vi "RunningAverage-AddResultChannels.vi"(8 "Error in":errorcluster, 10 "CD Settings in":T1 {"CD Task Dependency Ref" format="%.0x"; "CD Task Dependency" format="%.0x"}, 11 "Custom Device ref":T2 format="%.0x") -> (0 "Error out":errorcluster, 3 "Custom Device ref out":T2 format="%.0x")   [LabVIEW 2017, in "Waveform-Processing-Custom-Device Shared.lvlib" / "Running Average.lvlib"]
uses:
  Running Average.lvlib
  <vilib>/NI Veristand/Custom Device API/Custom Device Item Ref.ctl
  Custom Device Settings.ctl
  <vilib>/NI Veristand/Custom Device API/Custom Device Channel.ctl
  <vilib>/NI Veristand/Custom Device API/Custom Device Channel Type.ctl
  NationalInstruments.VeriStand.SystemStorage
  Constants.vi
  <vilib>/NI Veristand/Custom Device API/Get Item Property (Dependent Node Pointer).vi
  <vilib>/NI Veristand/Custom Device API/Set Item Property (Dependent Node Pointer).vi
  <vilib>/NI Veristand/Custom Device API/Custom Device API.lvlib
  Waveform-Processing-Custom-Device Shared.lvlib
  System Explorer/Waveform-Processing-Custom-Device System Explorer.lvlib
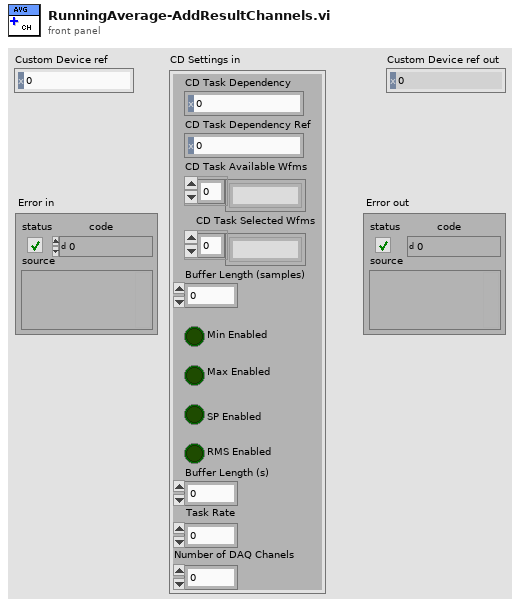
[diagram p1: front panel]
types:
  T1 = typedef "Waveform-Processing-Custom-Device Shared.lvlib/Custom Device Settings.ctl" = cluster{"CD Task Dependency":T2, "CD Task Dependency Ref":T2, "CD Task Available Wfms":string[], "CD Task Selected Wfms":string[], "Buffer Length (samples)":u32, "Min Enabled":bool, "Max Enabled ":bool, "SP Enabled":bool, "RMS Enabled":bool, "Buffer Length (s)":dbl, "Task Rate":dbl, "Number of DAQ Chanels":u32}
  T2 = typedef "Custom Device API.lvlib/Custom Device Item Ref.ctl" = u64
  T3 = typedef "Custom Device API.lvlib/Custom Device Channel Type.ctl" = enum16{"Input", "Output"}
  T4 = typedef "Custom Device API.lvlib/Custom Device Channel.ctl" = cluster{"Type":T3, "Units":string, "Default Value":dbl, "Faultable":bool, "Scalable":bool}
  T5 = cluster{"Waveform Name":string, "Units":string}[]
  T6 = typedef "Custom Device API.lvlib/Custom Device Pointer.ctl" = refnum<k24>
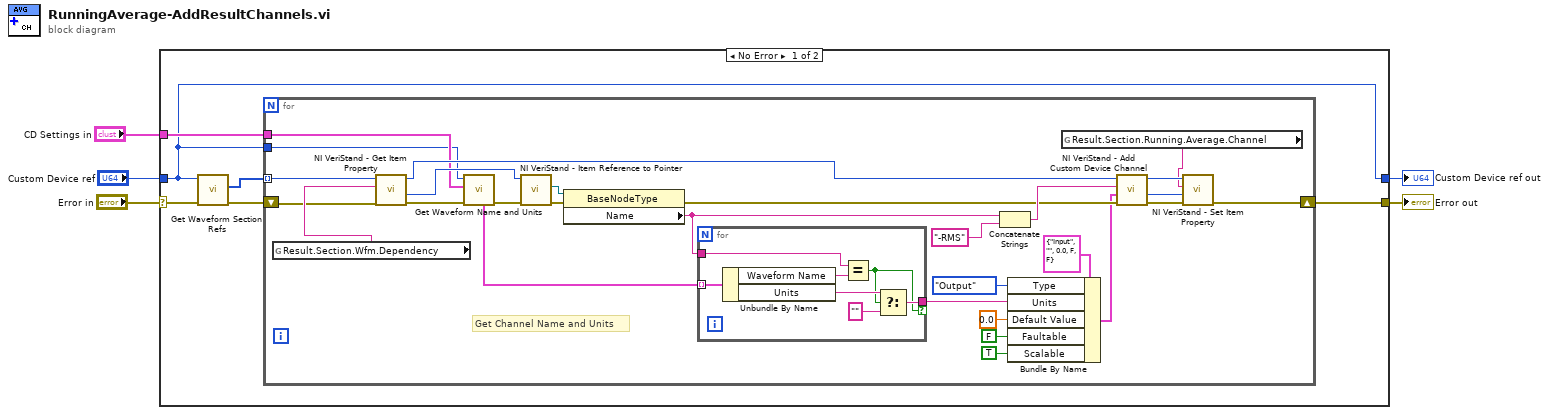
[diagram p0: block diagram]
diagram:
  n1 = case shown="No Error" "Error in" {
    selector: "Error in" -> [w11 w48]
    tunnel: "Custom Device ref" -> [w6 w47]
    tunnel: [w8 w48] -> w4
    tunnel: [w6 w47] -> w2
    tunnel: "CD Settings in" -> [w7 _]
    frame No Error {
      n2 = call "Get Waveform Section Refs.vi"("Error in"=w11, "Device Ref in"=w6) -> ("Error out"=w10:errorcluster, "Result Section Refs"=w9:T2[])  [unwired: 7 in, 1 out]
      n3 = for {
        tunnel: w9 -> [w34] mode=indexing
        shift-right: [w26] -> w8
        shift-left: w10 -> [w33]
        tunnel: w7 -> [w13]
        tunnel: w6 -> [w12]
        # "Get Channel Name and Units"
        n4 = global read "Constants.vi" "Result.Section.Wfm.Dependency"() -> (w39:string)
        n5 = call-poly <vilib>:"NI VeriStand - Get Item Property.vi"("error in (no error)"=w33, "Property Name"=w39, "Item Ref in"=w34) -> ("error out"=w24:errorcluster, "Dependent Node Ref"=w25:T2, "Item Ref out"=w38:T2)  [unwired: 5 in, 1 out]
        n6 = call "Get Waveform Name and Units.vi"("Error In"=w24, "CD Settings"=w13, "CustomDevice Ref"=w12) -> ("Error Out"=w23:errorcluster, "Waveform Channel Name and Units"=w15:T5)  [unwired: 7 in]
        n7 = call <vilib>:"NI VeriStand - Item Reference to Pointer.vi"("error in (no error)"=w23, "Item Ref in"=w25) -> ("error out"=w36:errorcluster, "Node Pointer"=w31:T6)  [unwired: 6 in, 2 out]
        n8 = property class="BaseNodeType"(reference=w31, error in=w36) -> (error out=w32:errorcluster, "Name"=w14:string)  [unwired: 1 out]
        n9 = for {
          tunnel: w15 -> [w45] mode=indexing
          tunnel: w14 -> [w46]
          tunnel: [w42] -> w16 if=w40
          n10 = Unbundle By Name(w45) -> ("Waveform Name"=w44:string, "Units"=w43:string)
          n11 = Equal?(x=w46, y=w44) -> (x = y?=w40:bool)
          n12 = Select(t=w43, s=w40, f="") -> (s? t:f=w42:string)
        }
        n13 = Concatenate Strings(w14, "-RMS" ("Property Name")) -> (w37:string)
        n14 = Bundle By Name(cluster=T4 {"Type"=enum."Input", "Units"="", "Default Value"=0.0, "Faultable"=FALSE, "Scalable"=FALSE} ("Channel"), "Type"=Custom_Device_Channel_Type."Output", "Units"=w16, "Default Value"=0.0, "Faultable"=FALSE, "Scalable"=TRUE) -> (w18:T4)
        n15 = global read "Constants.vi" "Result.Section.Running.Average.Channel"() -> (w28:string)
        n16 = call <vilib>:"NI VeriStand - Add Custom Device Channel.vi"("error in (no error)"=w32, "Channel"=w18, "Channel Name"=w37, "Parent Ref in"=w38) -> ("error out"=w27:errorcluster, "Channel Ref"=w29:T2, "Parent Ref out"=w30:T2)  [unwired: 4 in, 1 out]
        n17 = call-poly <vilib>:"NI VeriStand - Set Item Property.vi"("error in (no error)"=w27, "Dependent Node Ref"=w29, "Property Name"=w28, "Item Ref in"=w30) -> ("error out"=w26:errorcluster)  [unwired: 5 in, 2 out]
      }
    }
    frame Error {
    }
  }
  "Error out" <- w4
  "Custom Device ref out" <- w2
